vi "arithmetic.vi"() -> ()   [LabVIEW 2018]
panel:
  out "x / y":dbl
  out "x * y":dbl
  out "x - y":dbl
  out "x + y":dbl
  in  "숫자형 2":dbl
  in  "숫자형":dbl
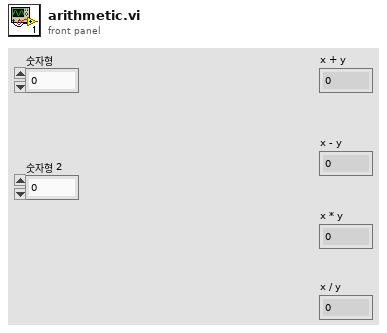
[diagram p1: front panel]
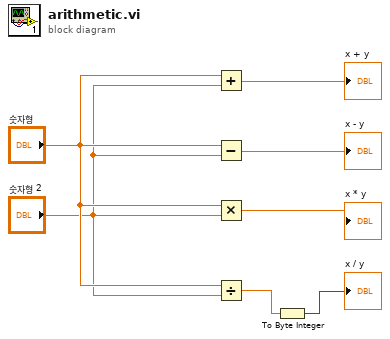
[diagram p0: block diagram]
diagram:
  n1 = Add(x="숫자형", y="숫자형 2") -> (x+y=→"x + y":dbl)
  n2 = Subtract(x="숫자형", y="숫자형 2") -> (x-y=→"x - y":dbl)
  n3 = Multiply(x="숫자형", y="숫자형 2") -> (x*y=→"x * y":dbl)
  n4 = Divide(x="숫자형", y="숫자형 2") -> (x/y=w2:dbl)
  n5 = To Byte Integer(number=w2) -> (8bit integer=→"x / y":i8)
